vi "CRC32Test.vi"() -> ()   [LabVIEW 2016]
uses:
  FPGA/CRC32/CRC32Settings.ctl
  <vilib>/rvi/Emulation/niFpgaEmulationIsFPGAContextNoSignature.vi
  <vilib>/rvi/Emulation/niFpgaSctlEmulationGetInTimedLoop.vi
  <vilib>/rvi/errors/niFpgaSetErrorForExecOnDevCompSimple.vi
  <vilib>/rvi/eio/common/nirviEmuReportErrorAndStop.vi
  <vilib>/rvi/DataTransferAndStorage/Container/Common/niFpgaContainerGetUniqueNameForEmu.vi
  <vilib>/rvi/FIFO/Fifo_Resource/nirvififoEmulationSetSize.vi
  <vilib>/rvi/FIFO/Fifo_Resource/nirviFifoEmulationQueueMgr.vi
  <instcachedir>/0/nirviFifoEmulationQueueMgr_E5CAEC123FF24DC58D834DCA3CDAA9B5.lvgen/nirviFifoEmulationQueueMgr_E5CAEC123FF24DC58D834DCA3CDAA9B5_009.vi
  <vilib>/rvi/FIFO/Fifo_Resource/nirvififoEmulationDetermineInputValidOut.vi
  <vilib>/rvi/FIFO/Fifo_Resource/nirvififoEmulationCreateLock.vi
  <vilib>/rvi/Emulation/niFpgaProcessEmulError.vi
  <vilib>/rvi/FIFO/Fifo_Resource/nirvififoEmulationObtainLock.vi
  <vilib>/rvi/FIFO/Fifo_Resource/nirvififoEmulationReleaseLock.vi
  <vilib>/rvi/occurrence/nirviWaitOnOccurrenceBase.vi
  <vilib>/rvi/errors/nirviReportUnexpectedCaseInternalError.vi
  <vilib>/rvi/errors/nirviReportUnexpectedCaseInternalError (U32).vi
  <instcachedir>/0/nirviFifoEmulationQueueMgr_E5CAEC123FF24DC58D834DCA3CDAA9B5.lvgen/nirviFifoEmulationQueueMgr_E5CAEC123FF24DC58D834DCA3CDAA9B5_004.vi
  <instcachedir>/0/nirviFifoEmulationQueueMgr_E5CAEC123FF24DC58D834DCA3CDAA9B5.lvgen/nirviFifoEmulationQueueMgr_E5CAEC123FF24DC58D834DCA3CDAA9B5_006.vi
  <vilib>/Utility/error.llb/Clear Errors.vi
  <vilib>/rvi/DataTransferAndStorage/Container/XNode/niFpgaContainer.xnode
  <vilib>/rvi/FIFO/Fifo_Resource/nirvififoEmulationWrite.vi
  <vilib>/rvi/FIFO/Fifo_Resource/nirvififoEmulationRead.vi
panel:
  out "CRC":u32 format="%08x"
  in  "Size":i32=32
  in  "Input":u8[](array[numeric])=[254, 129, 255, 85, 128, 0, 0, 0, 128, 0, 0, 0, 52, 186, 110, 247, 128, 0, 0, 0, 128, 0, 0, 0, 128, 0, 0, 0, 4, 5, 0, 36, 0, 0, 0, 0, 0, 0, 0, 0, 0, 0, 0, 0, 0, 0, 0, 0, 0, 0, 0, 0, 0, 0, 0, 0, 0, 0, 0, 0, 0, 0, 0, 0, 0, 0, 0, 0, 0, 0, 0, 0, 0, 0, 0, 0, 0, 0, 0, 0, 0, 0, 0, 0, 0, 0, 0, 0, 0, 0, 0, 0, 0, 0, 0, 0, 0, 0, 0, 0, 0, 0, 0, 0, 0, 0, 0, 0, 0, 0, 0, 0, 0, 0, 0, 0, 0, 0, 0, 0, 0, 0, 0, 0, 0, 0, 0, 0] format="%02x"
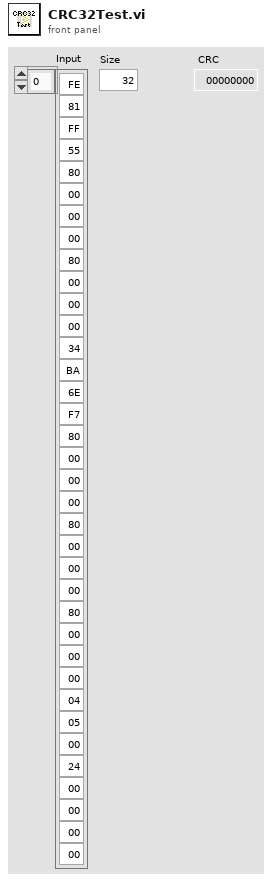
[diagram p1: front panel]
types:
  T1 = typedef "CRC32Settings.ctl" = cluster{"DataFIFO":refnum<k21>, "CalculateFIFO":refnum<k21>, "CRCFIFO":refnum<k21>}
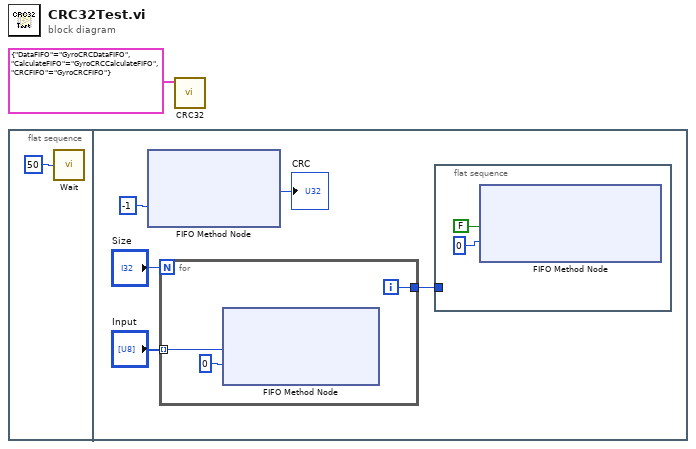
[diagram p0: block diagram]
diagram:
  n1 = flat-sequence {
    frame #0 {
      n2 = call "Wait"("Count(uSec)"=u32 50) -> ()  [unwired: 1 out]
    }
    frame #1 {
      n3 = xnode ("FIFO Method Node")("Timeout"=-1) -> ("Element"=→"CRC":u32)  [unwired: 1 in, 2 out]
      n4 = for {
        N: "Size" -> [_]
        tunnel: "Input" -> [w10] mode=indexing
        tunnel: [w12] -> w5
        i -> [w12]
        n5 = xnode ("FIFO Method Node")("Element"=w10, "Timeout"=0) -> ()  [unwired: 1 in, 2 out]
      }
      n6 = flat-sequence {
        tunnel: w5 -> [_]
        frame #0 {
          n7 = xnode ("FIFO Method Node")("Element"=FALSE, "Timeout"=0) -> ()  [unwired: 1 in, 2 out]
        }
      }
    }
  }
  n8 = call "CRC32.vi"("CRC32Settings"=T1 {"DataFIFO"="GyroCRCDataFIFO", "CalculateFIFO"="GyroCRCCalculateFIFO", "CRCFIFO"="GyroCRCFIFO"}) -> ()  [unwired: 11 in]
